vi "Pre Launch Init.vi"(11 "PLC_Module in":refnum<class "PLC_Module.lvclass">) -> (0 "error out":errorcluster, 3 "PLC_Module out":refnum<class "PLC_Module.lvclass">)   [LabVIEW 2025, in "PLC_Module.lvlib" / "PLC_Module.lvclass"]
doc: "<p>(<strong>Filename</strong>: <span class=\"dnl\">Actor Framework.lvlib:Actor.lvclass:Pre Launch Init.vi</span>)</p>\n<p>Defines behavior that occurs after the <a href=\"nihelplauncher://docs/csh?context=lvcore_lvcomm_af_launch_nested_actor\">Launch Nested Actor</a> method is invoked but before the actor's Actor Core method begins running.</p>\n<p>By default, this method does nothing. A descendant class may override it to define behavior.</p>"
uses:
  PLC_Module.lvclass
  PLC_Module.lvclass/PLC_Module.ctl
  Module/Module/Module/Module.lvclass
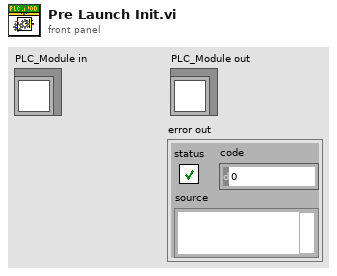
[diagram p1: front panel]
types:
  T1 = typedef "PLC_Module.lvlib/PLC_Module.lvclass/PLC_Connect_Config.ctl" = cluster{"IP Address":string, "Port":u16, "Timeout":i32}
  T2 = typedef "PLC_Module.lvlib/PLC_Module.lvclass/PLC_Data_Config.ctl" = map{string, cluster{"Config":T3, "Get Value":string, "Set Value":string}}
  T3 = typedef "PLC_Module.lvlib/PLC_Module.lvclass/PLC_Data.ctl" = cluster{"Address":string, "Direction":enum16{"PC->PLC", "PLC->PC"}, "DataType":T4, "Description":string}
  T4 = typedef "PLC_Module.lvlib/PLC_Module.lvclass/PLC_Data_Type.ctl" = enum16{"Boolean", "Single Float", "U8", "U32", "U32_Array", "String"}
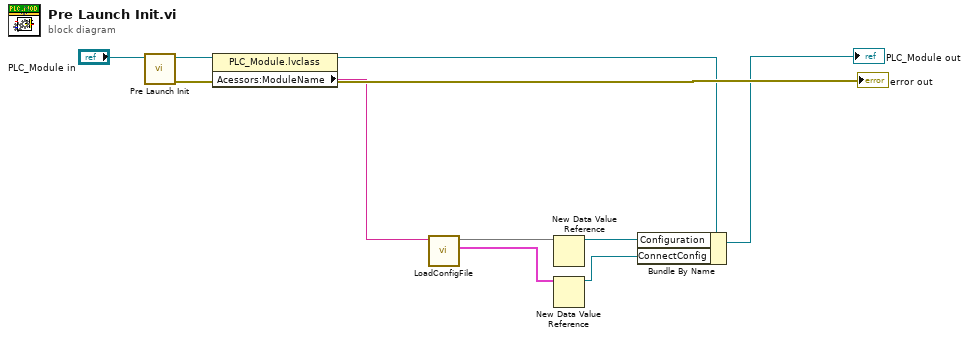
[diagram p0: block diagram]
diagram:
  n1 = call-parent "Pre Launch Init.vi"("Module in"="PLC_Module in") -> ("error out"=→"error out":errorcluster, "Module out"=w8:refnum<class "PLC_Module.lvclass">)  [unwired: 9 in]
  n2 = property class="PLC_Module.lvclass"(reference=w8) -> (reference out=w4:refnum<class "PLC_Module.lvclass">, "Acessors:ModuleName"=w3:string)  [unwired: 1 in, 1 out]
  n3 = call "LoadConfigFile.vi"("Model Name"=w3) -> ("ConnectConfig"=w2:T1, "Data out"=w5:T2)  [unwired: 7 in, 2 out]
  n4 = New Data Value Reference(data value=w5) -> (data value reference=w7:refnum<data-value>)  [unwired: 1 in, 1 out]
  n5 = New Data Value Reference(data value=w2) -> (data value reference=w1:refnum<data-value>)  [unwired: 1 in, 1 out]
  n6 = Bundle By Name(cluster=w4, "Configuration"=w7, "ConnectConfig"=w1) -> (→"PLC_Module out":refnum<class "PLC_Module.lvclass">)
